vi "ALTS-2015 Update Status Light Indicator.vi"(7 "DO Options":T1, 8 "error in":errorcluster, 11 "Station Cluster":T2) -> (0 "error out":errorcluster)   [LabVIEW 2013]
uses:
  Controls/ALTS-2015 Station Cluster.ctl
  Controls/ALTS-2015 Digital Output Options.ctl
  SLL DAQ Engine/Software/Source Code/Sub VIs/DAQ Engine/Controls/SLL DE DO Global Options.ctl
  SLL DAQ Engine/Software/Source Code/Sub VIs/DAQ Engine/Controls/SLL DE List of Digital Outputs.ctl
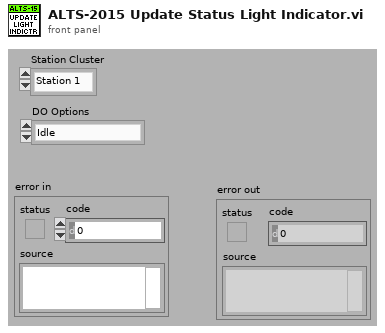
[diagram p1: front panel]
types:
  T1 = typedef "ALTS-2015 Digital Output Options.ctl" = enum16{"Idle", "Test Running", "Pass", "Fail"}
  T2 = typedef "ALTS-2015 Station Cluster.ctl" = enum16{"Station 1", "Station 2", "Station 3", "Station 4"}
  T3 = typedef "SLL DE DO Global Options.ctl" = enum16{"Init", "Write Line", "Write Array", "Write Full Status", "Read Line", "Read Array", "Read Full Status", "Restart DO", "Send to Safe Mode", "Stop DO"}
  T4 = typedef "SLL DE List of Digital Outputs.ctl" = enum16{"STATION1_START TEST", "STATION1_STOP TEST", "STATION1_LIGHT1", "STATION1_LIGHT2", "STATION1_LIGHT3", "STATION1_SELECT_TEST", "STATION2_START TEST", "STATION2_STOP TEST", "STATION2_LIGHT1", "STATION2_LIGHT2", "STATION2_LIGHT3", "STATION2_SELECT_TEST", "STATION3_START TEST", "STATION3_STOP TEST", "STATION3_LIGHT1", "STATION3_LIGHT2", "STATION3_LIGHT3", "STATION3_SELECT_TEST", "STATION4_START TEST", "STATION4_STOP TEST", "STATION4_LIGHT1", "STATION4_LIGHT2", "STATION4_LIGHT3", "STATION4_SELECT_TEST"}
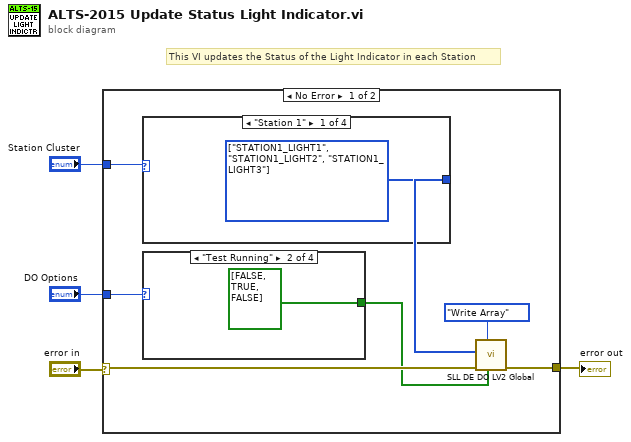
[diagram p0: block diagram]
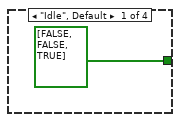
[diagram p2: hidden frame]
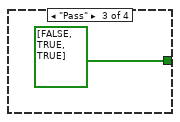
[diagram p3: hidden frame]
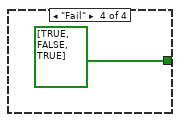
[diagram p4: hidden frame]
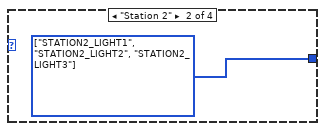
[diagram p5: hidden frame]
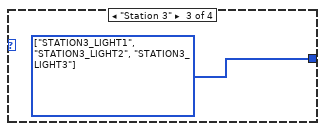
[diagram p6: hidden frame]
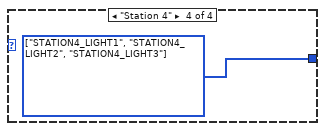
[diagram p7: hidden frame]
diagram:
  # "This VI updates the Status of the Light Indicator in each Station"
  n1 = case shown="No Error" "error in" {
    selector: "error in" -> [w9 w20]
    tunnel: "DO Options" -> [w6 _]
    tunnel: [w8 w20] -> w4
    tunnel: "Station Cluster" -> [w11 _]
    frame No Error {
      n2 = case shown="\"Station 1\"" w11 {
        tunnel: [w16 w17 w18 w19] -> w7
        frame "Station 1" {
          w16 = T4[] [enum."STATION1_LIGHT1", enum."STATION1_LIGHT2", enum."STATION1_LIGHT3"] items=["STATION1_START TEST", "STATION1_STOP TEST", "STATION1_LIGHT1", "STATION1_LIGHT2", "STATION1_LIGHT3", "STATION1_SELECT_TEST", "STATION2_START TEST", "STATION2_STOP TEST", "STATION2_LIGHT1", "STATION2_LIGHT2", "STATION2_LIGHT3", "STATION2_SELECT_TEST", "STATION3_START TEST", "STATION3_STOP TEST", "STATION3_LIGHT1", "STATION3_LIGHT2", "STATION3_LIGHT3", "STATION3_SELECT_TEST", "STATION4_START TEST", "STATION4_STOP TEST", "STATION4_LIGHT1", "STATION4_LIGHT2", "STATION4_LIGHT3", "STATION4_SELECT_TEST"] ("DO Channel Name Array")
        }
        frame "Station 2" {
          w17 = T4[] [enum."STATION2_LIGHT1", enum."STATION2_LIGHT2", enum."STATION2_LIGHT3"] items=["STATION1_START TEST", "STATION1_STOP TEST", "STATION1_LIGHT1", "STATION1_LIGHT2", "STATION1_LIGHT3", "STATION1_SELECT_TEST", "STATION2_START TEST", "STATION2_STOP TEST", "STATION2_LIGHT1", "STATION2_LIGHT2", "STATION2_LIGHT3", "STATION2_SELECT_TEST", "STATION3_START TEST", "STATION3_STOP TEST", "STATION3_LIGHT1", "STATION3_LIGHT2", "STATION3_LIGHT3", "STATION3_SELECT_TEST", "STATION4_START TEST", "STATION4_STOP TEST", "STATION4_LIGHT1", "STATION4_LIGHT2", "STATION4_LIGHT3", "STATION4_SELECT_TEST"] ("DO Channel Name Array")
        }
        frame "Station 3" {
          w18 = T4[] [enum."STATION3_LIGHT1", enum."STATION3_LIGHT2", enum."STATION3_LIGHT3"] items=["STATION1_START TEST", "STATION1_STOP TEST", "STATION1_LIGHT1", "STATION1_LIGHT2", "STATION1_LIGHT3", "STATION1_SELECT_TEST", "STATION2_START TEST", "STATION2_STOP TEST", "STATION2_LIGHT1", "STATION2_LIGHT2", "STATION2_LIGHT3", "STATION2_SELECT_TEST", "STATION3_START TEST", "STATION3_STOP TEST", "STATION3_LIGHT1", "STATION3_LIGHT2", "STATION3_LIGHT3", "STATION3_SELECT_TEST", "STATION4_START TEST", "STATION4_STOP TEST", "STATION4_LIGHT1", "STATION4_LIGHT2", "STATION4_LIGHT3", "STATION4_SELECT_TEST"] ("DO Channel Name Array")
        }
        frame "Station 4" {
          w19 = T4[] [enum."STATION4_LIGHT1", enum."STATION4_LIGHT2", enum."STATION4_LIGHT3"] items=["STATION1_START TEST", "STATION1_STOP TEST", "STATION1_LIGHT1", "STATION1_LIGHT2", "STATION1_LIGHT3", "STATION1_SELECT_TEST", "STATION2_START TEST", "STATION2_STOP TEST", "STATION2_LIGHT1", "STATION2_LIGHT2", "STATION2_LIGHT3", "STATION2_SELECT_TEST", "STATION3_START TEST", "STATION3_STOP TEST", "STATION3_LIGHT1", "STATION3_LIGHT2", "STATION3_LIGHT3", "STATION3_SELECT_TEST", "STATION4_START TEST", "STATION4_STOP TEST", "STATION4_LIGHT1", "STATION4_LIGHT2", "STATION4_LIGHT3", "STATION4_SELECT_TEST"] ("DO Channel Name Array")
        }
      }
      n3 = case shown="\"Test Running\"" w6 {
        tunnel: [bool[] [FALSE, FALSE, TRUE] ("DO State Array") bool[] [FALSE, TRUE, FALSE] ("DO State Array") bool[] [FALSE, TRUE, TRUE] ("DO State Array") bool[] [TRUE, FALSE, TRUE] ("DO State Array")] -> w5
        frame "Idle", Default {
        }
        frame "Test Running" {
        }
        frame "Pass" {
        }
        frame "Fail" {
        }
      }
      n4 = call "SLL DE DO LV2 Global.vi"("DO State Array"=w5, "DO Option"=SLL_DE_DO_Global_Options."Write Array", "Error In"=w9, "DO Channel Name Array"=w7) -> ("error out"=w8:errorcluster)  [unwired: 4 in, 3 out]
    }
    frame Error {
    }
  }
  "error out" <- w4
